vi "Measure.vi"(6 "Graph in":cluster{dbl[], dbl[]}, 8 "error in":errorcluster, 10 "Reference Cell":i32) -> (0 "error out":errorcluster, 1 "Values":cluster{dbl[], dbl[]}, 2 "P1/P2":dbl format="%#_13g")   [LabVIEW 2013]
uses:
  GlobalVariables/AllowContinuousPressureAcquisition.vi
  GlobalVariables/ValveParameters.vi
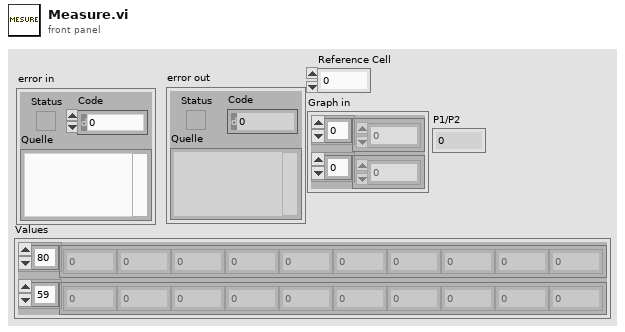
[diagram p1: front panel]
types:
  T1 = cluster{"baudrate":u32, "databits":u16, "paritybit":u16, "stopbits":u16, "flux control":u16, "Port":string, "Serial Parameters":cluster{"Mode":enum16{"RTU", "ASCII"}, "Slave Address":u8}, "Timeout":u32, "Valve mapping":cluster{"Inlet Valve":u8, "V1":u8, "V2":u8, "Sample Valve":u8, "Outlet Valve":u8}}
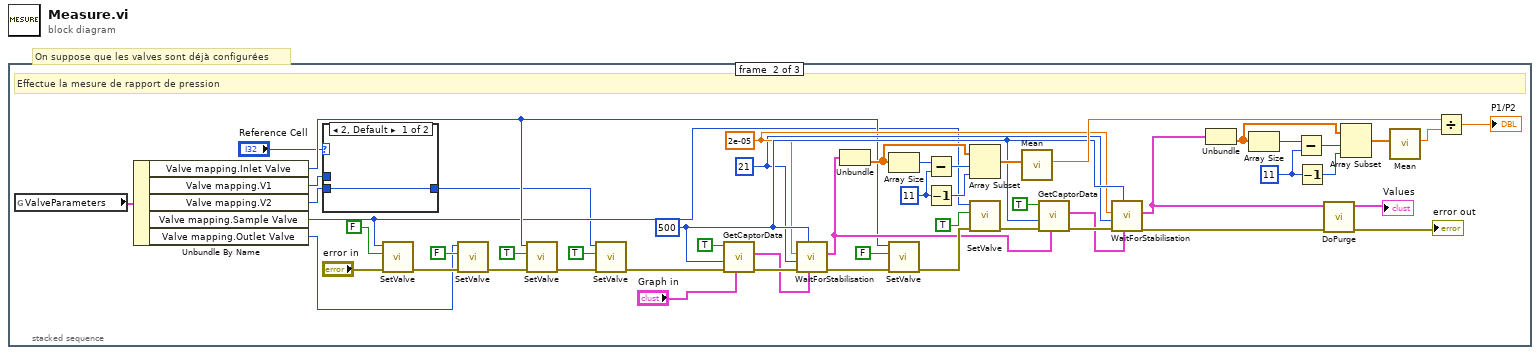
[diagram p0: block diagram]
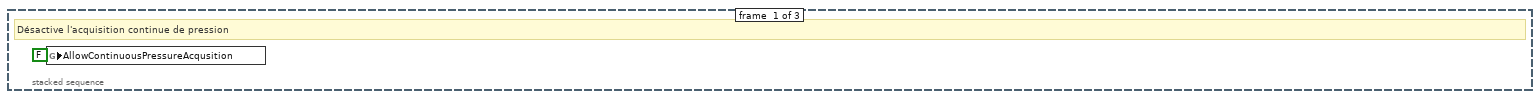
[diagram p2: hidden frame]
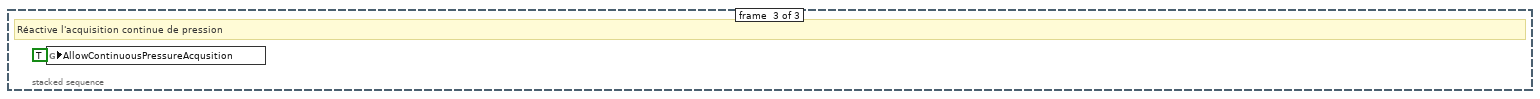
[diagram p4: hidden frame]
diagram:
  # "On suppose que les valves sont déjà configurées"
  n1 = stacked-sequence {
    frame #0 {
      # "Désactive l'acquisition continue de pression"
      n2 = global write "AllowContinuousPressureAcquisition.vi" "AllowContinuousPressureAcqusition"(FALSE) -> ()
    }
    frame #1 {
      w16 = 500
      w15 = 2e-05
      w14 = 21
      w35 = 11
      w40 = 11
      # "Effectue la mesure de rapport de pression"
      n3 = global read "ValveParameters.vi" "ValveParameters"() -> (w13:T1)
      n4 = Unbundle By Name(w13) -> ("Valve mapping.Inlet Valve"=w12:u8, "Valve mapping.V1"=w8:u8, "Valve mapping.V2"=w7:u8, "Valve mapping.Sample Valve"=w11:u8, "Valve mapping.Outlet Valve"=w10:u8)
      n5 = case shown="2, Default" "Reference Cell" {
        tunnel: w8 -> [_ w55]
        tunnel: w7 -> [w54 _]
        tunnel: [w54 w55] -> w6
        frame 2, Default {
        }
        frame 1 {
        }
      }
      n6 = call "SetValve.vi"("error in"="error in", "ON"=FALSE, "Valve"=w11) -> ("error out"=w29:errorcluster)  [unwired: 8 in]
      n7 = call "SetValve.vi"("error in"=w29, "ON"=FALSE, "Valve"=w10) -> ("error out"=w51:errorcluster)  [unwired: 8 in]
      n8 = call "SetValve.vi"("error in"=w51, "ON"=TRUE, "Valve"=w12) -> ("error out"=w49:errorcluster)  [unwired: 8 in]
      n9 = call "SetValve.vi"("error in"=w49, "ON"=TRUE, "Valve"=w6) -> ("error out"=w24:errorcluster)  [unwired: 8 in]
      n10 = call "GetCaptorData.vi"("Graph in"="Graph in", "error in"=w24, "Length"=w16, "ON"=TRUE) -> ("error out"=w22:errorcluster, "Values"=w20:cluster{dbl[], dbl[]})  [unwired: 6 in]
      n11 = call "WaitForStabilisation.vi"("Graph in"=w20, "WaitTime"=w16, "error in"=w22, "SampleCount"=w14, "Variance/Mean Trigger"=w15) -> ("error out"=w21:errorcluster, "Values"=w19:cluster{dbl[], dbl[]})  [unwired: 5 in]
      n12 = Unbundle(w19) -> (w44:dbl[])  [unwired: 1 out]
      n13 = Array Size(array=w44) -> (size(s)=w43:i32)
      n14 = call "SetValve.vi"("error in"=w21, "ON"=FALSE, "Valve"=w12) -> ("error out"=w47:errorcluster)  [unwired: 8 in]
      n15 = Subtract(x=w43, y=w40) -> (x-y=w42:i32)
      n16 = Decrement(x=w40) -> (x-1=w41:i32)
      n17 = Array Subset(array=w44, index=w42, length=w41) -> (w31:dbl[])
      n18 = call "SetValve.vi"("error in"=w47, "ON"=TRUE, "Valve"=w11) -> ("error out"=w26:errorcluster)  [unwired: 8 in]
      n19 = call "Mean.vi"("Array"=w31) -> ("Mean"=w32:dbl)  [unwired: 10 in]
      n20 = call "GetCaptorData.vi"("Graph in"=w19, "error in"=w26, "Length"=w16, "ON"=TRUE) -> ("error out"=w18:errorcluster, "Values"=w17:cluster{dbl[], dbl[]})  [unwired: 6 in]
      n21 = call "WaitForStabilisation.vi"("Graph in"=w17, "WaitTime"=w16, "error in"=w18, "SampleCount"=w14, "Variance/Mean Trigger"=w15) -> ("error out"=w4:errorcluster, "Values"=w3:cluster{dbl[], dbl[]})  [unwired: 5 in]
      n22 = Unbundle(w3) -> (w39:dbl[])  [unwired: 1 out]
      n23 = Array Size(array=w39) -> (size(s)=w38:i32)
      n24 = Subtract(x=w38, y=w35) -> (x-y=w37:i32)
      n25 = Decrement(x=w35) -> (x-1=w36:i32)
      n26 = call "DoPurge.vi"("error in (no error)"=w4, "Graph in"=w3) -> ("error out"=→"error out":errorcluster, "Values"=→"Values":cluster{dbl[], dbl[]})  [unwired: 8 in]
      n27 = Array Subset(array=w39, index=w37, length=w36) -> (w34:dbl[])
      n28 = call "Mean.vi"("Array"=w34) -> ("Mean"=w33:dbl)  [unwired: 10 in]
      n29 = Divide(x=w32, y=w33) -> (x/y=→"P1/P2":dbl)
    }
    frame #2 {
      # "Réactive l'acquisition continue de pression"
      n30 = global write "AllowContinuousPressureAcquisition.vi" "AllowContinuousPressureAcqusition"(TRUE) -> ()
    }
  }
